vi "获取默认流程路径.vi"(7 "复合步骤":bool, 11 "参数":string[](array[string])) -> (3 "路径":path)   [LabVIEW 2016, in "斯坦道通用流路CODmn.lvlib"]
uses:
  <vilib>/Utility/sysdir.llb/System Directory Type.ctl
  <vilib>/regexp/Match Regular Expression.xnode
panel:
  out "正则表达式":string
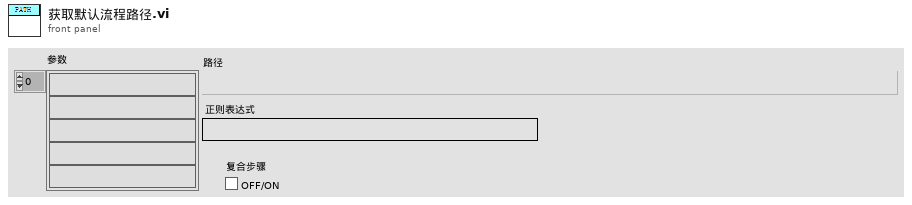
[diagram p1: front panel]
types:
  T1 = typedef "System Directory Type.ctl" = i32
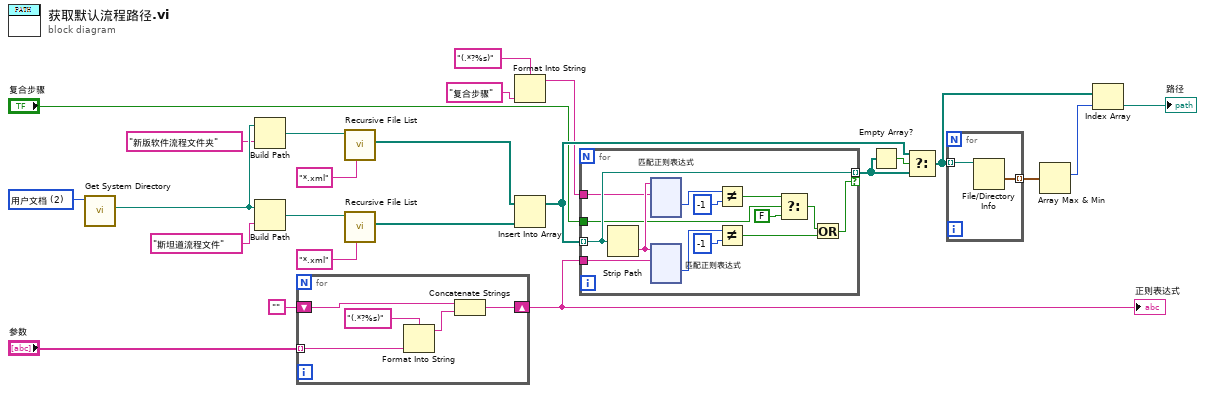
[diagram p0: block diagram]
diagram:
  w8 = T1 2 items=["用户目录"=0, "用户桌面"=1, "用户文档"=2, "用户应用程序数据"=3, "用户设置"=4, "用户临时目录"=5, "公共文档"=6, "公共应用程序数据"=7, "公共设置"=8, "公共缓存"=13, "系统核心库"=9, "系统安装库"=10, "应用程序文件"=11, "启动盘根目录"=12] ("system directory type")
  n1 = call <vilib>:"Get System Directory.vi"("system directory type"=w8) -> ("system directory"=w12:path)  [unwired: 10 in]
  n2 = Build Path(base path=w12, name or relative path="新版软件流程文件夹" ("名称或相对路径")) -> (appended path=w11:path)
  n3 = Build Path(base path=w12, name or relative path="斯坦道流程文件" ("名称或相对路径")) -> (appended path=w15:path)
  n4 = for {
    tunnel: "参数" -> [w29] mode=indexing
    shift-right: [w26] -> w5
    shift-left: "" -> [w25]
    n5 = Format Into String(format string="(.*?%s)" ("格式字符串"), w29) -> (resulting string=w27:string)  [unwired: 2 in, 1 out]
    n6 = Concatenate Strings(w25, w27) -> (w26:string)
  }
  "正则表达式" <- w5
  n7 = call <vilib>:"Recursive File List.vi"("pattern"="*.xml", "Folder Path"=w11) -> ("All Files in Dir"=w16:path[])  [unwired: 5 in, 4 out]
  n8 = call <vilib>:"Recursive File List.vi"("pattern"="*.xml", "Folder Path"=w15) -> ("All Files in Dir"=w17:path[])  [unwired: 5 in, 4 out]
  n9 = Format Into String(format string="(.*?%s)" ("格式字符串"), "复合步骤" ("输入 1")) -> (resulting string=w2:string)  [unwired: 2 in, 1 out]
  n10 = Insert Into Array(array=w16, new element=w17) -> (w22:path[])  [unwired: 1 in]
  n11 = for {
    tunnel: w22 -> [w42] mode=indexing
    tunnel: w5 -> [w43]
    tunnel: [w42] -> w23 mode=indexing if=w34
    tunnel: w2 -> [w37]
    tunnel: "复合步骤" -> [w33]
    n12 = Strip Path(path=w42) -> (name=w38:string)  [unwired: 1 out]
    n13 = xnode "匹配正则表达式"("输入字符串"=w38, "正则表达式"=w37) -> ("匹配后偏移量"=w35:i32)  [unwired: 4 in, 4 out]
    n14 = xnode "匹配正则表达式"("输入字符串"=w38, "正则表达式"=w43) -> ("匹配后偏移量"=w41:i32)  [unwired: 4 in, 4 out]
    n15 = Not Equal?(x=w35, y=-1) -> (x != y?=w32:bool)
    n16 = Not Equal?(x=w41, y=-1) -> (x != y?=w39:bool)
    n17 = Select(t=w32, s=w33, f=FALSE) -> (s? t:f=w31:bool)
    n18 = Or(x=w31, y=w39) -> (x .or. y?=w34:bool)
  }
  n19 = Empty Array?(array=w23) -> (empty?=w21:bool)
  n20 = Select(t=w22, s=w21, f=w23) -> (s? t:f=w24:path[])
  n21 = for {
    tunnel: w24 -> [w272] mode=indexing
    tunnel: [w273] -> w19 mode=indexing
    n22 = File/Directory Info(path=w272) -> (last mod=w273:timestamp)  [unwired: 1 in, 6 out]
  }
  n23 = Array Max & Min(array=w19) -> (max index (indices)=w18:i32)  [unwired: 3 out]
  n24 = Index Array(array=w24, index=w18) -> (element=→"路径":path)
